vi "ZAlign_Search_Locals.vi"(8 "error in (no error)":errorcluster, 10 "Ctrls[]":refnum<vi>[](array[refnum]), 11 "Controls[]":refnum<vi>[](array[refnum])) -> (0 "error out":errorcluster, 3 "Array":refnum<vi>[](array[refnum]))   [LabVIEW 2014, in "ZAlign.lvlib"]
doc: "ZAlign.lvlib:ZAlign_Search_Locals.vi\n----------------------------------------------\nSearch Local controls\n\nInputs:\n---------------------\n- error in (no error) : Cluster; \n- Ctrls[] : 1DArrayOfRefnum; \n- Controls[] : 1DArrayOfRefnum; \n\nOutputs:\n---------------------\n- error out : Cluster; \n- Array : 1DArrayOfRefnum; \n\n----------------------------------------------\n16/03/2015\nZühlke Engineering AG\nCH-8952 Schlieren\nwww.zuehlke.com"
uses:
  ZAlign.lvlib
panel:
  # "Connector Pane"
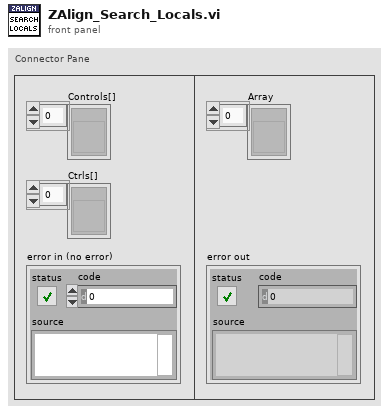
[diagram p1: front panel]
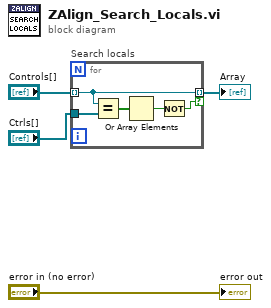
[diagram p0: block diagram]
diagram:
  n1 = for "Search locals" {
    tunnel: "Controls[]" -> [w7] mode=indexing
    tunnel: "Ctrls[]" -> [w9]
    tunnel: [w7] -> w4 mode=indexing if=w5
    n2 = Equal?(x=w7, y=w9) -> (x = y?=w8:bool[])
    n3 = Or Array Elements(Boolean array=w8) -> (logical OR=w6:bool)
    n4 = Not(x=w6) -> (.not. x?=w5:bool)
  }
  "Array" <- w4
  "error out" <- "error in (no error)"
